vi "DarkStar_V4_LabJack.vi"() -> ()   [LabVIEW 2020]
doc: "This example shows how to use the Write to Spreadsheet VI to write data to a Comma Separated Value (CSV) spreadsheet file which can be read in Microsoft Excel."
uses:
  <vilib>/Analysis/baseanly.llb/Mean (DBL).vi
  <vilib>/Utility/file.llb/Write Delimited Spreadsheet (string).vi
  <vilib>/Utility/file.llb/Write Delimited Spreadsheet (DBL).vi
  <vilib>/Analysis/NI_AALBase.lvlib
panel:
  out "Fuel Injector Pressure":dbl(graph)
  out "Error String":string
  out "error out":errorcluster
  out "Chamber Pressure":dbl[][](graph)
  out "Thrust":dbl[][](graph)
  out "LOX Injector Pressure":dbl[][](graph)
  out "Write Headers":bool
  in  "Folder Path":string="C:\\Users\\Griffin\\Desktop\\"
  out "File Path String":string
  in  "Log Data":bool
  in  "Scan Stop":bool
  out "SampleRate (Hz)":dbl format="%.3f"
  in  "STREAM_RESOLUTION_INDEX":i32
  in  "STREAM_SETTLING_US":i32
  out "ScansPerRead":i32
  out "# of iterations":i32
  out "LJMScanBacklog":i32
  out "DeviceScanBacklog":i32
  out "Error Message":string
  in  "Scan Rate (Hz)":dbl=100.0 format="%.3f"
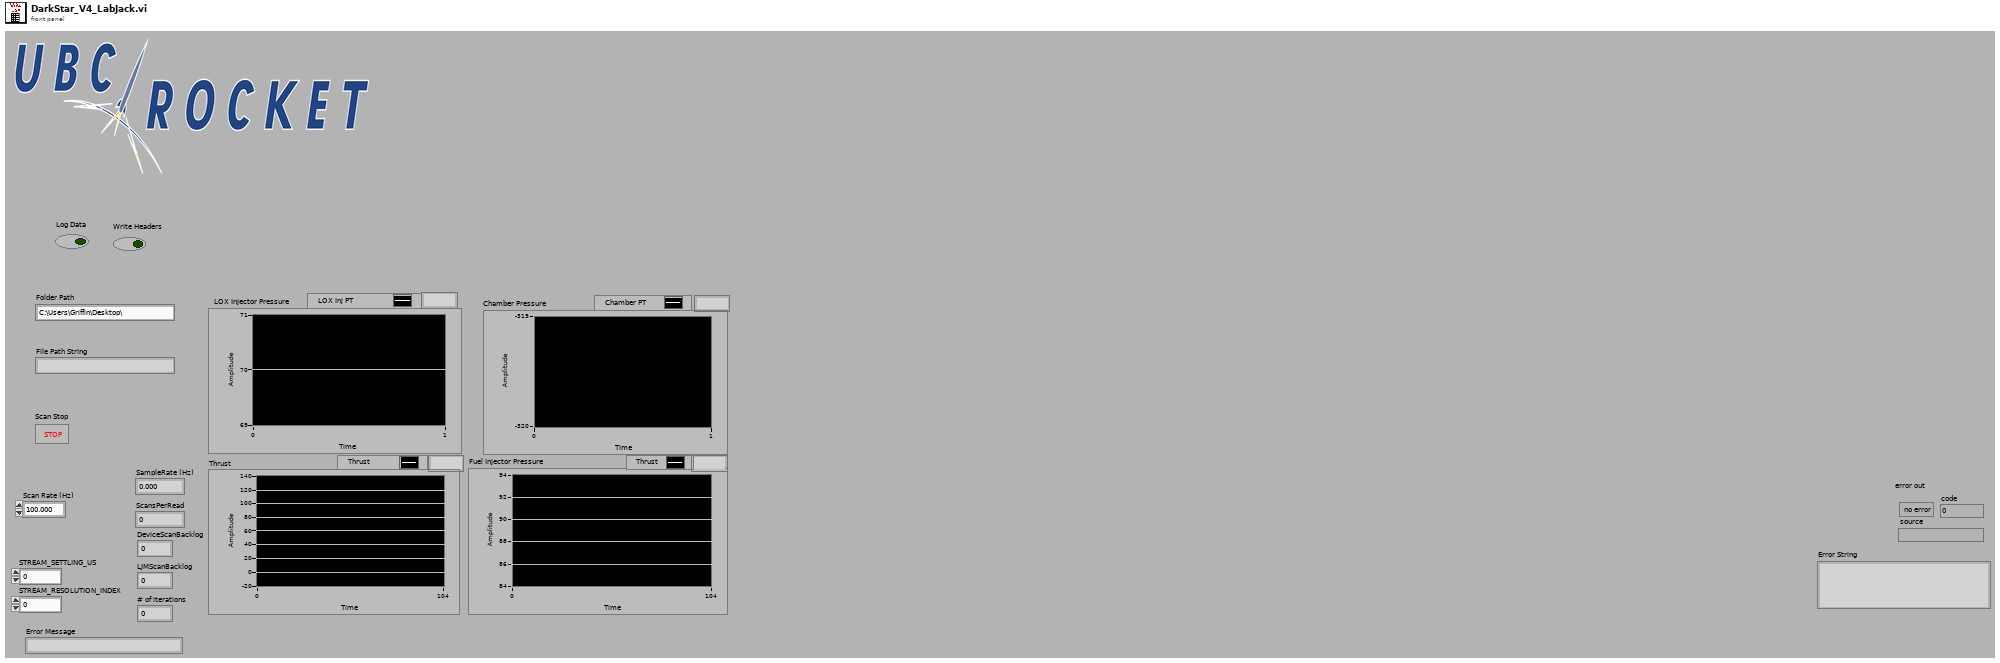
[diagram p1: front panel]
types:
  T1 = typedef "NI_Matrix.lvlib/RealMatrix.ctl" = dbl[][]
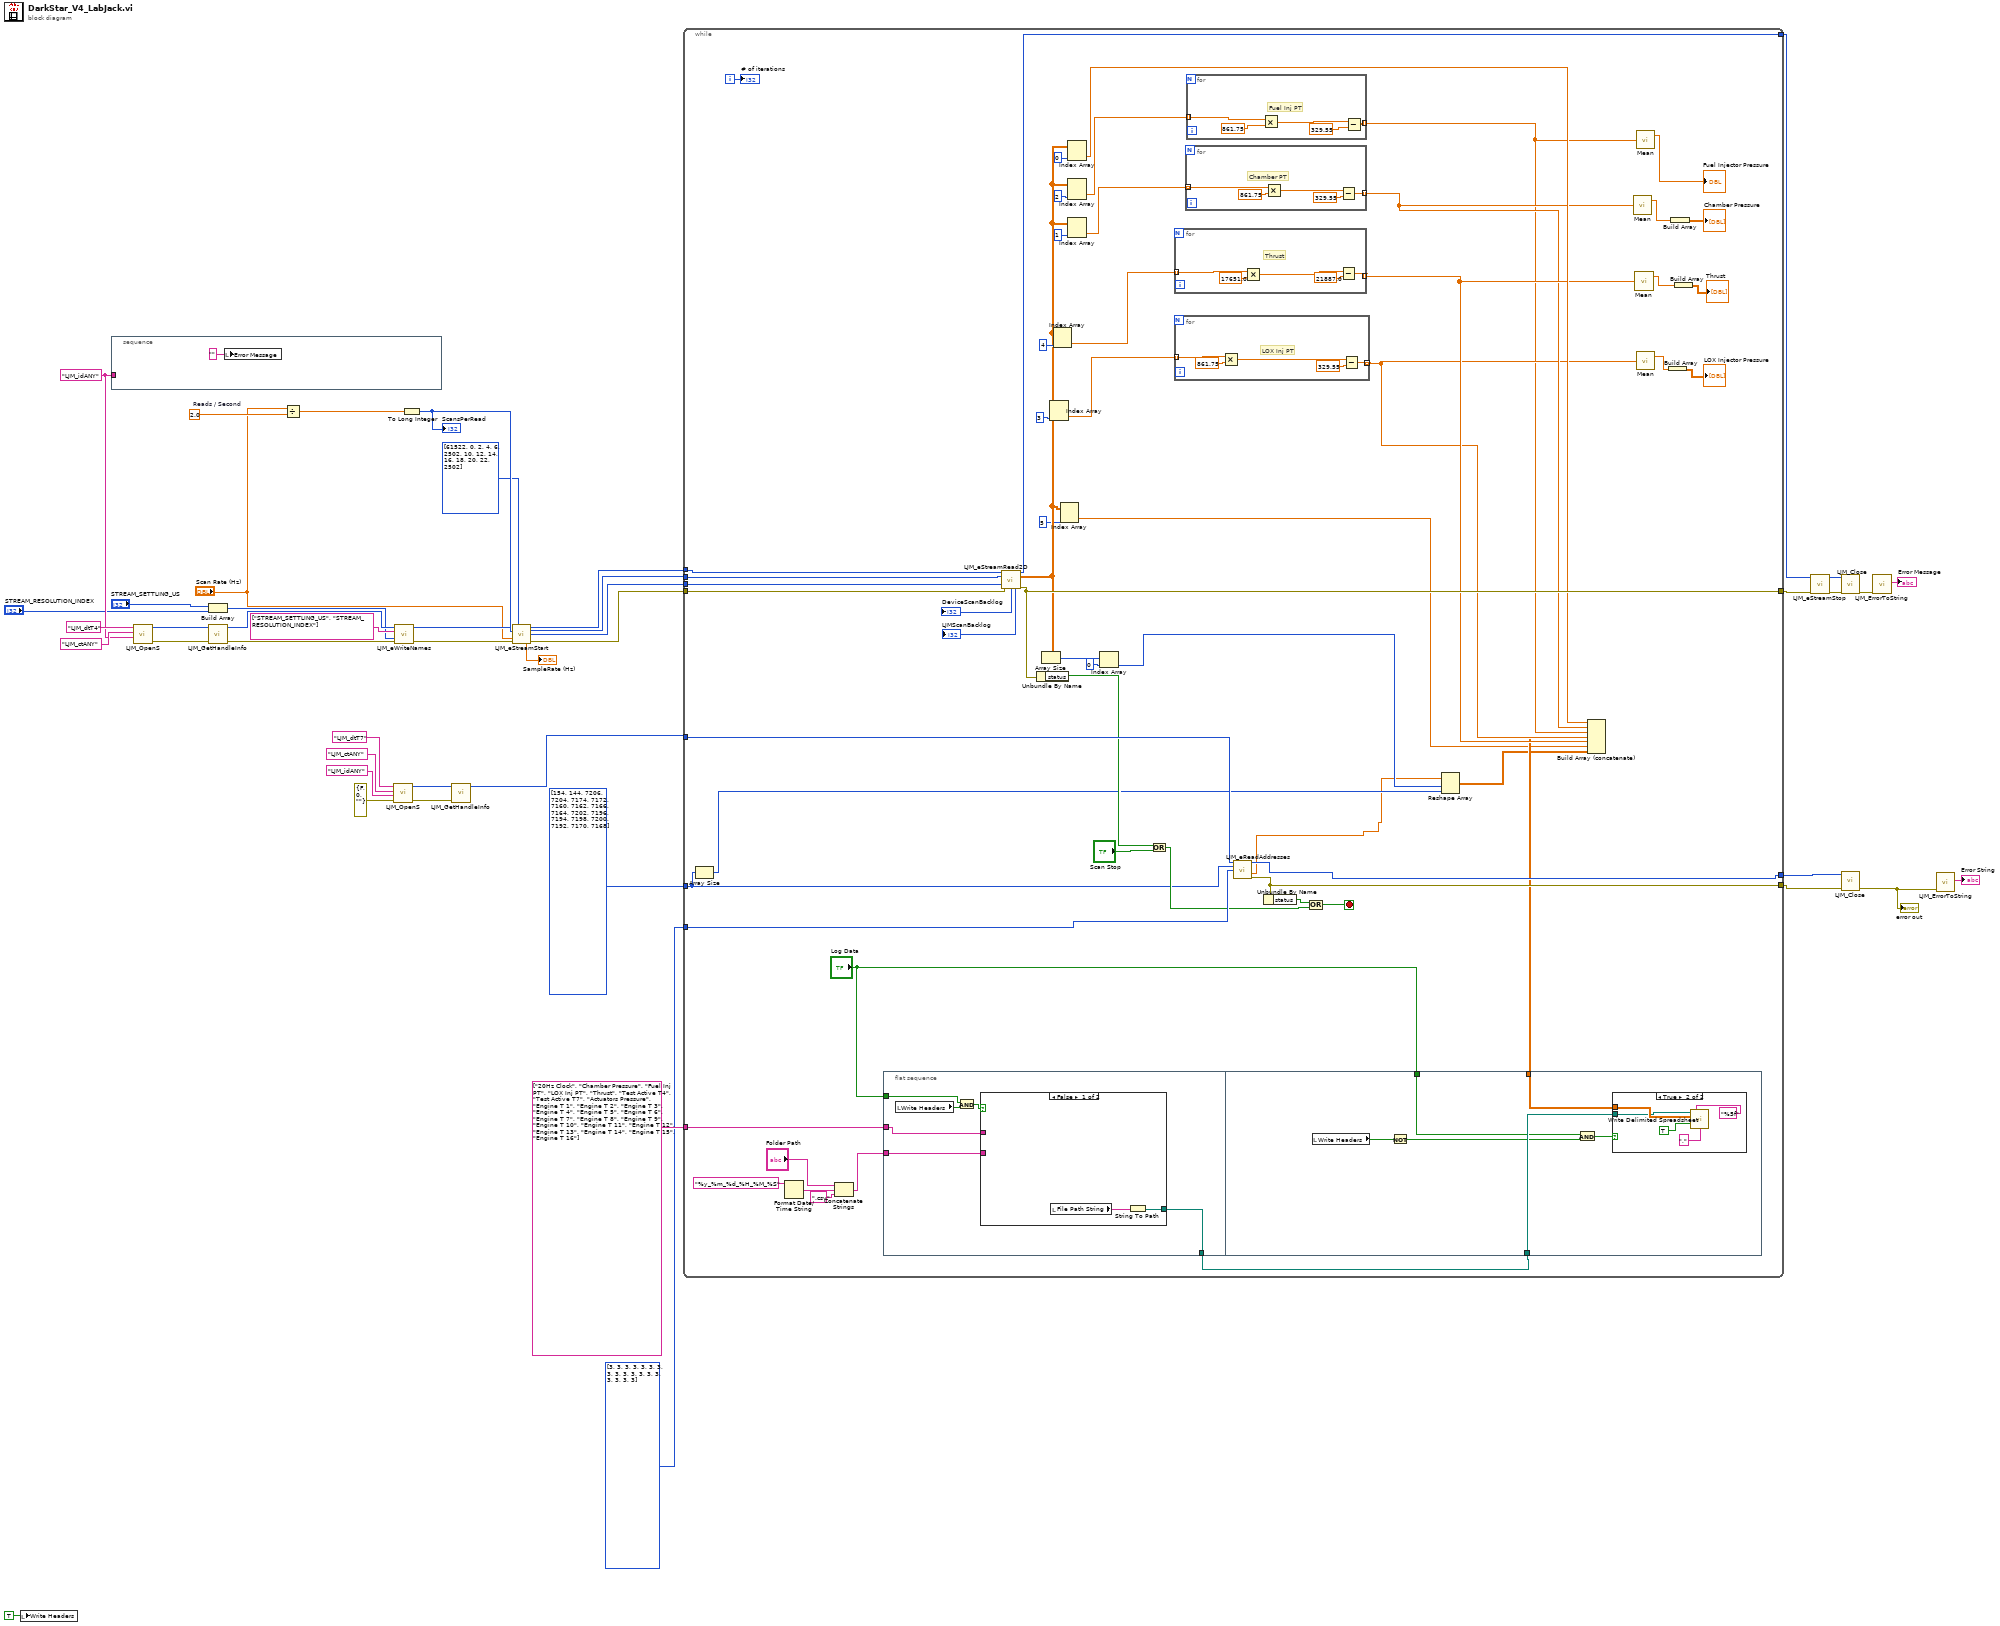
[diagram p0: block diagram]
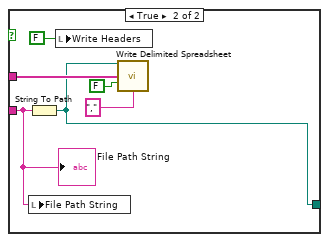
[diagram p2: hidden frame]
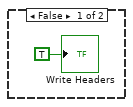
[diagram p3: hidden frame]
diagram:
  w32 = "LJM_idANY" ("Identifier")
  w31 = 2.0  # Reads / Second
  n1 = local write "Write Headers"(TRUE ("Write Headers")) -> ()
  n2 = stacked-sequence {
    tunnel: w32 -> [_]
    frame #0 {
      n3 = local write "Error Message"("" ("Error Message")) -> ()
    }
  }
  n4 = call "LJM_OpenS.vi"("Identifier"=w32, "ConnectionType"="LJM_ctANY", "DeviceType"="LJM_dtT4") -> ("error out"=w36:errorcluster, "Handle"=w33:i32)  [unwired: 7 in]
  n5 = Build Array("STREAM_SETTLING_US", "STREAM_RESOLUTION_INDEX") -> (w24:i32[])
  n6 = call "LJM_GetHandleInfo.vi"("error in"=w36, "Handle In"=w33) -> ("error out"=w28:errorcluster, "Handle Out"=w27:i32)  [unwired: 2 in, 6 out]
  n7 = Divide(x="Scan Rate (Hz)", y=w31) -> (x/y=w30:dbl)
  n8 = call "LJM_OpenS.vi"("error in"=errorcluster {"status"=FALSE, "code"=0, "source"=""} ("error in (no error)"), "Identifier"="LJM_idANY", "ConnectionType"="LJM_ctANY", "DeviceType"="LJM_dtT7") -> ("error out"=w12:errorcluster, "Handle"=w11:i32)  [unwired: 6 in]
  n9 = call "LJM_eWriteNames.vi"("Handle In"=w27, "aNames"=string[] ["STREAM_SETTLING_US", "STREAM_RESOLUTION_INDEX"], "aValuesIn"=w24, "error in"=w28) -> ("Handle Out"=w26:i32, "error out"=w21:errorcluster)  [unwired: 9 in, 1 out]
  n10 = To Long Integer(number=w30) -> (32bit integer=w29:i32)
  "ScansPerRead" <- w29
  n11 = call "LJM_GetHandleInfo.vi"("error in"=w12, "Handle In"=w11) -> ("Handle Out"=w5:i32)  [unwired: 2 in, 7 out]
  n12 = call "LJM_eStreamStart.vi"("Handle In"=w26, "aScanList"=i32[] [61522, 0, 2, 4, 6, 2502, 10, 12, 14, 16, 18, 20, 22, 2502] ("Modbus Scan List"), "ScansPerRead"=w29, "ScanRate"="Scan Rate (Hz)", "error in"=w21) -> ("Handle Out"=w43:i32, "ScansPerRead Out"=w18:i32, "NumReadAddresses"=w19:i32, "Actual SampleRate"=→"SampleRate (Hz)":dbl, "error out"=w44:errorcluster)  [unwired: 5 in, 1 out]
  n13 = while {
    tunnel: [w101] -> w41
    tunnel: w43 -> [w87]
    tunnel: w19 -> [w97]
    tunnel: w18 -> [w96]
    tunnel: w44 -> [w102]
    tunnel: [w98] -> w42
    tunnel: string[] ["20Hz Clock", "Chamber Pressure", "Fuel Inj PT", "LOX Inj PT", "Thrust", "Test Active T4", "Test Active T7", "Actuators Pressure", "Engine T 1", "Engine T 2", "Engine T 3", "Engine T 4", "Engine T 5", "Engine T 6", "Engine T 7", "Engine T 8", "Engine T 9", "Engine T 10", "Engine T 11", "Engine T 12", "Engine T 13", "Engine T 14", "Engine T 15", "Engine T 16"] -> [w77]
    tunnel: i32[] [3, 3, 3, 3, 3, 3, 3, 3, 3, 3, 3, 3, 3, 3, 3, 3, 3, 3] ("aTypes") -> [w67]
    tunnel: i32[] [154, 144, 7206, 7204, 7174, 7172, 7160, 7162, 7166, 7164, 7202, 7196, 7194, 7198, 7200, 7192, 7170, 7168] ("aAddresses") -> [w48]
    tunnel: w5 -> [w66]
    tunnel: [w65] -> w2
    tunnel: [w64] -> w1
    i -> [w103]
    stop <- w60 stop-if-true
    n14 = Array Size(array=w48) -> (size(s)=w56:i32)
    n15 = Format Date/Time String(time format string (%c)="%y_%m_%d_%H_%M_%S") -> (date/time string=w82:string)  [unwired: 2 in]
    n16 = Concatenate Strings("Folder Path", w82, ".csv" ("string")) -> (w79:string)
    n17 = flat-sequence {
      tunnel: w77 -> [w109]
      tunnel: w79 -> [w108]
      tunnel: [w107] -> w46
      tunnel: "Log Data" -> [w106]
      tunnel: w59 -> [w123]
      tunnel: w46 -> [w122]
      tunnel: "Log Data" -> [w119]
      frame #0 {
        n18 = local read "Write Headers"() -> (w104:bool)
        n19 = And(x=w106, y=w104) -> (x .and. y?=w105:bool)
        n20 = case shown="False" w105 {
          tunnel: w109 -> [_ w117]
          tunnel: [w110 w114] -> w107
          tunnel: w108 -> [_ w113]
          frame False {
            n21 = local read "File Path String"() -> (w111:string)
            n22 = String To Path(string=w111) -> (path=w110:path)
          }
          frame True {
            n23 = String To Path(string=w113) -> (path=w114:path)
            n24 = local write "File Path String"(w113) -> ()
            n25 = local write "Write Headers"(FALSE) -> ()
            n26 = call-poly <vilib>:"Write Delimited Spreadsheet.vi"("file path (dialog if empty)"=w114, "1D data"=w117, "append to file? (new file:F)"=FALSE, "delimiter (\\t)"="," ("delimiter (\\t)")) -> ()  [unwired: 10 in, 2 out]
            "File Path String" <- w113
          }
        }
      }
      frame #1 {
        n27 = local read "Write Headers"() -> (w121:bool)
        n28 = Not(x=w121) -> (.not. x?=w120:bool)
        n29 = And(x=w119, y=w120) -> (x .and. y?=w118:bool)
        n30 = case shown="True" w118 {
          tunnel: w123 -> [_ w127]
          tunnel: w122 -> [_ w126]
          frame False {
            "Write Headers" <- TRUE ("Write Headers")
          }
          frame True {
            n31 = call-poly <vilib>:"Write Delimited Spreadsheet.vi"("file path (dialog if empty)"=w126, "format (%.3f)"="%5f", "2D data"=w127, "append to file? (new file:F)"=TRUE, "delimiter (\\t)"="," ("delimiter (\\t)")) -> ()  [unwired: 9 in, 2 out]
          }
        }
      }
    }
    n32 = call "LJM_eStreamRead2D.vi"("Handle In"=w87, "ScansPerRead"=w96, "NumAddresses"=w97, "error in"=w102) -> ("Handle Out"=w101:i32, "aData Out"=w51:dbl[][], "DeviceScanBacklog"=→"DeviceScanBacklog":i32, "LJMScanBacklog"=→"LJMScanBacklog":i32, "error out"=w98:errorcluster)  [unwired: 7 in]
    n33 = Unbundle By Name(w98) -> ("status"=w62:bool)
    n34 = Array Size(array=w51) -> (size(s)=w57:i32[])
    n35 = Index Array(array=w51, index (col)=3) -> (element=w90:dbl[])  [unwired: 1 in]
    n36 = Index Array(array=w51, index (col)=4) -> (element=w85:dbl[])  [unwired: 1 in]
    n37 = Index Array(array=w51, index (col)=5) -> (element=w49:dbl[])  [unwired: 1 in]
    n38 = Index Array(array=w51, index (col)=0) -> (element=w86:dbl[])  [unwired: 1 in]
    n39 = Index Array(array=w51, index (col)=2) -> (element=w92:dbl[])  [unwired: 1 in]
    n40 = Index Array(array=w51, index (col)=1 ("disabled index (col)")) -> (element=w94:dbl[])  [unwired: 1 in]
    n41 = Index Array(array=w57, index=0) -> (element=w54:i32)
    n42 = Or(x=w62, y="Scan Stop") -> (x .or. y?=w61:bool)
    n43 = for {
      tunnel: w85 -> [w134] mode=indexing
      tunnel: [w130] -> w73 mode=indexing
      # "Thrust"
      n44 = Multiply(x=w134, y=17651.0) -> (x*y=w131:dbl)
      n45 = Subtract(x=w131, y=21887.0) -> (x-y=w130:dbl)
    }
    n46 = for {
      tunnel: w90 -> [w139] mode=indexing
      tunnel: [w136] -> w69 mode=indexing
      # "LOX Inj PT"
      n47 = Multiply(x=w139, y=861.75) -> (x*y=w135:dbl)
      n48 = Subtract(x=w135, y=329.55) -> (x-y=w136:dbl)
    }
    n49 = for {
      tunnel: w94 -> [w149] mode=indexing
      tunnel: [w145] -> w72 mode=indexing
      # "Chamber PT"
      n50 = Multiply(x=w149, y=861.75) -> (x*y=w147:dbl)
      n51 = Subtract(x=w147, y=329.55) -> (x-y=w145:dbl)
    }
    n52 = for {
      tunnel: w92 -> [w144] mode=indexing
      tunnel: [w142] -> w53 mode=indexing
      # "Fuel Inj PT"
      n53 = Multiply(x=w144, y=861.75) -> (x*y=w141:dbl)
      n54 = Subtract(x=w141, y=329.55) -> (x-y=w142:dbl)
    }
    n55 = call "LJM_eReadAddresses.vi"("Handle In"=w66, "aAddresses"=w48, "aTypes"=w67) -> ("Handle Out"=w65:i32, "aValues"=w47:dbl[], "error out"=w64:errorcluster)  [unwired: 9 in, 1 out]
    n56 = Unbundle By Name(w64) -> ("status"=w63:bool)
    n57 = Or(x=w63, y=w61) -> (x .or. y?=w60:bool)
    n58 = Reshape Array(w47, w54, w56) -> (w55:dbl[][])
    n59 = Build Array (concatenate)(w86, w72, w53, w69, w73, w49, w55) -> (w59:T1)
    n60 = call-poly <vilib>:"Mean.vi"("X"=w72) -> ("mean"=w71:dbl)  [unwired: 1 out]
    n61 = call-poly <vilib>:"Mean.vi"("X"=w73) -> ("mean"=w74:dbl)  [unwired: 1 out]
    n62 = call-poly <vilib>:"Mean.vi"("X"=w53) -> ("mean"=→"Fuel Injector Pressure":dbl)  [unwired: 1 out]
    n63 = call-poly <vilib>:"Mean.vi"("X"=w69) -> ("mean"=w70:dbl)  [unwired: 1 out]
    n64 = Build Array(w70) -> (→"LOX Injector Pressure":T1)
    n65 = Build Array(w71) -> (→"Chamber Pressure":T1)
    n66 = Build Array(w74) -> (→"Thrust":T1)
    "# of iterations" <- w103
  }
  n67 = call "LJM_eStreamStop.vi"("Handle In"=w41, "error in"=w42) -> ("Handle Out"=w39:i32, "error out"=w40:errorcluster)  [unwired: 12 in]
  n68 = call "LJM_Close.vi"("error in"=w40, "Handle"=w39) -> ("error out"=w38:errorcluster)  [unwired: 9 in]
  n69 = call "LJM_Close.vi"("error in"=w1, "Handle"=w2) -> ("error out"=w4:errorcluster)  [unwired: 9 in]
  "error out" <- w4
  n70 = call "LJM_ErrorToString.vi"("error in"=w38) -> ("String"=→"Error Message":string)  [unwired: 10 in]
  n71 = call "LJM_ErrorToString.vi"("error in"=w4) -> ("String"=→"Error String":string)  [unwired: 10 in]
